vi "Upgrade Component Dependencies.vi"(0 "NIPKG_LV in":refnum<class "NIPKG_LV.lvclass">, 11 "error in (no error)":errorcluster) -> (4 "NIPKG_LV out":refnum<class "NIPKG_LV.lvclass">, 15 "error out":errorcluster)   [LabVIEW 2017, in "CL_G3_VIComponentBuilder.lvlib" / "NIPKG_LV.lvclass"]
doc: "Upgrades the NI Package versions that this NI Packages depends on. Adds the upgraded version information to the release notes."
uses:
  NIPKG_LV.lvclass
  C:/Tool Chain Support/Software Module Builder/Source/Exports/NI Build Specification_LV/NI Build Specification_LV.lvclass
  C:/Tool Chain Support/Software Module Builder/Source/Exports/Exports/Export.lvclass
  NI Build Specification_LV/NI Build Specification_LV.lvclass/NI Build Specification_LV.ctl
  <userlib>/_Cirrus Logic/NI Package Manager API/Source/Version Comparison Operator.ctl
  <vilib>/Utility/error.llb/whitespace.ctl
  Exports/Export.lvclass/Export.ctl
  NI Build Specification_LV/Accessors/Read Project Reference.vi
  NI Build Specification_LV/Accessors/Read Build Spec Ref.vi
  Exports/Accessors/Write Export Operation Errors.vi
  <userlib>/_Cirrus Logic/NI Package Manager API/Source/TCS_NIPKG_API.lvlib
  <userlib>/_Cirrus Logic/NI Package Manager BldSpec Utils/Source/NIPKG BuildSpec API.lvlib
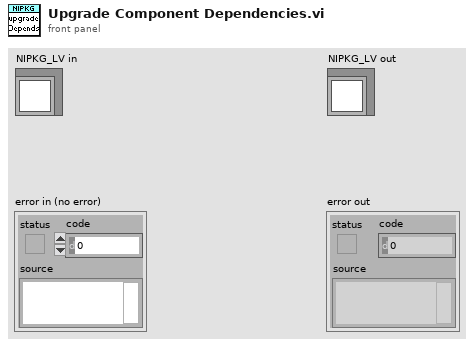
[diagram p1: front panel]
types:
  T1 = cluster{"NIPKG_LV":refnum<class "NIPKG_LV.lvclass">, "Upgrade Info":string[], "Release Notes":string, "Errors":errorcluster, "Release Notes Tag Name":string}
  T2 = typedef "TCS_NIPKG_API.lvlib/Version Comparison Operator.ctl" = enum16{">", ">=", "=", "!=", "<=", "<"}
  T3 = typedef "whitespace.ctl" = u16
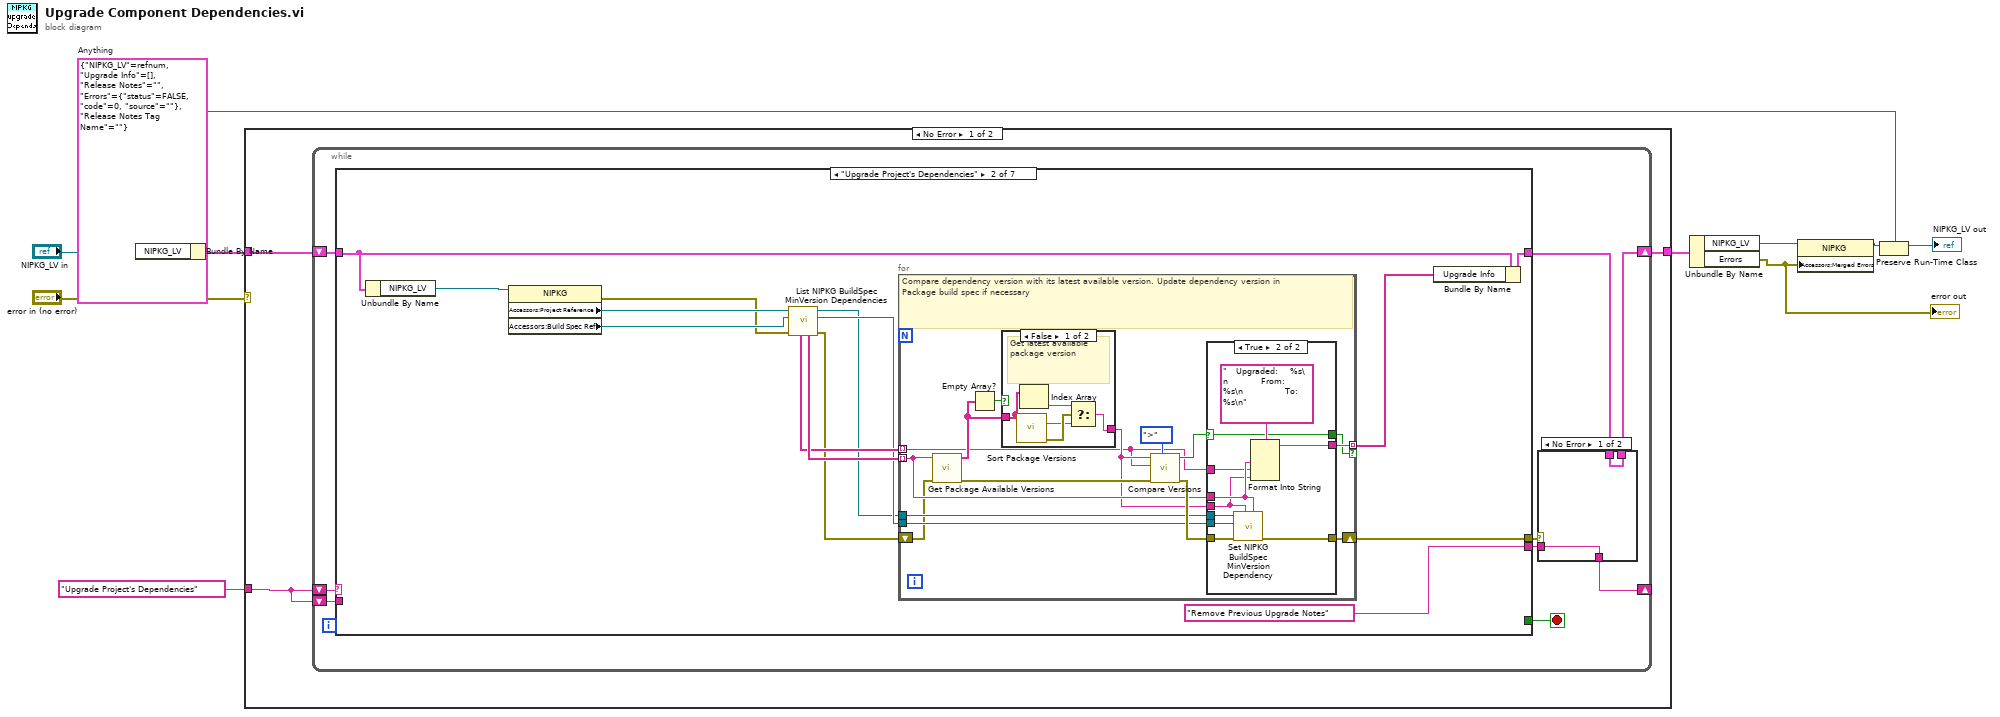
[diagram p0: block diagram]
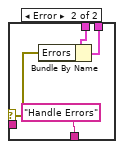
[diagram p2: hidden frame]
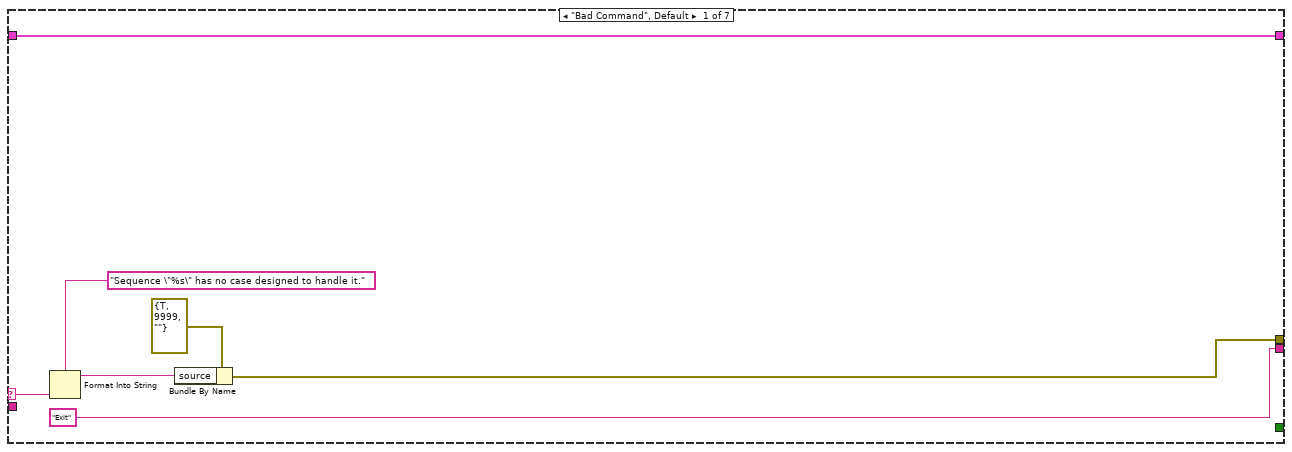
[diagram p3: hidden frame]
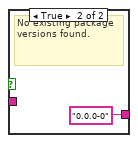
[diagram p4: hidden frame]
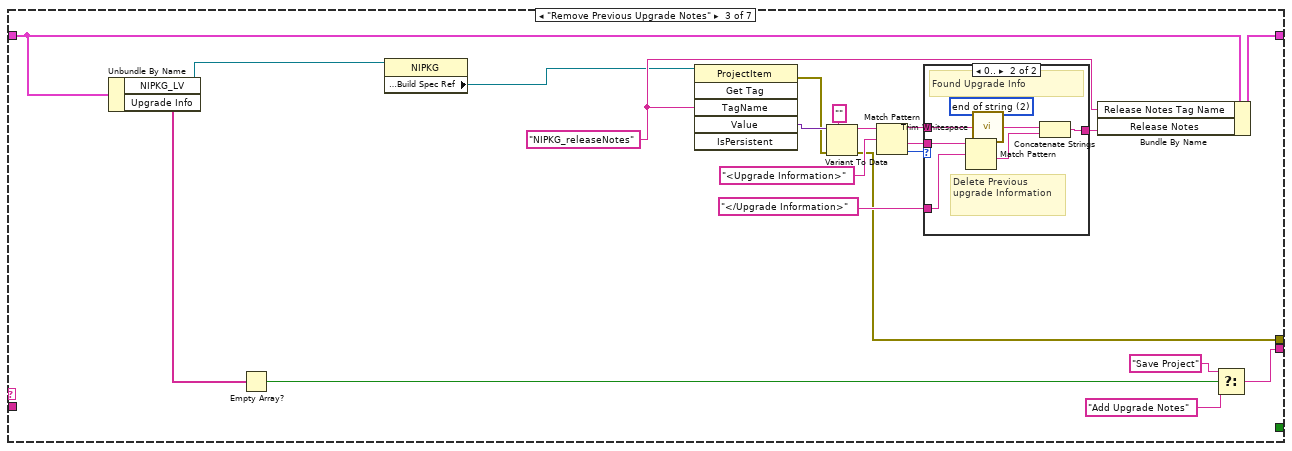
[diagram p6: hidden frame]
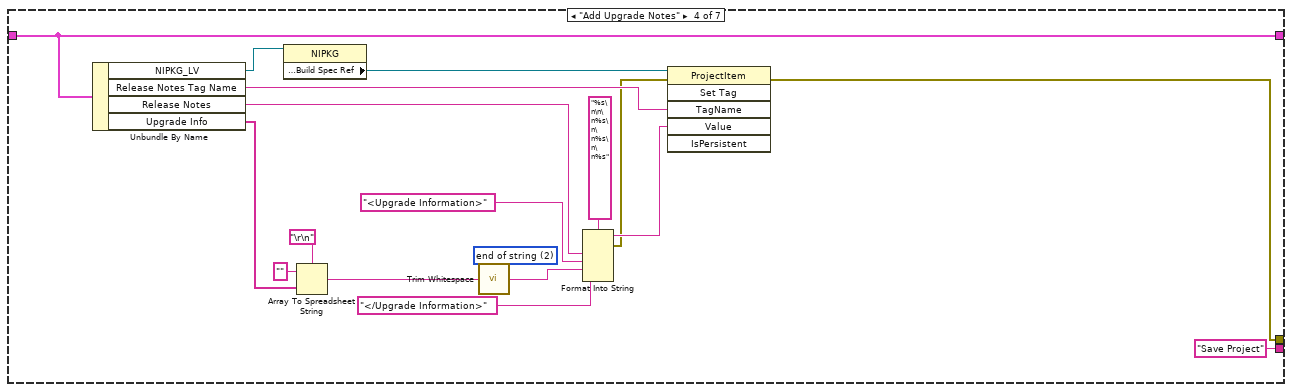
[diagram p8: hidden frame]
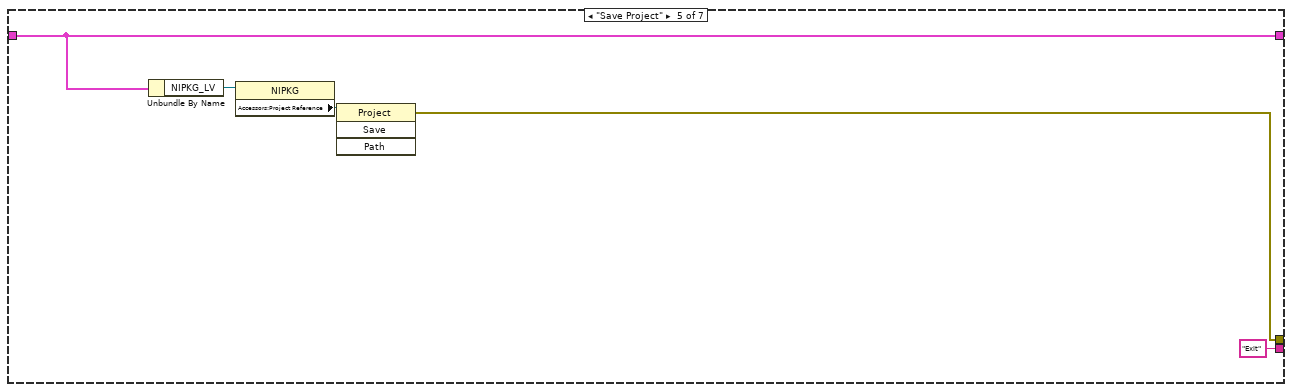
[diagram p9: hidden frame]
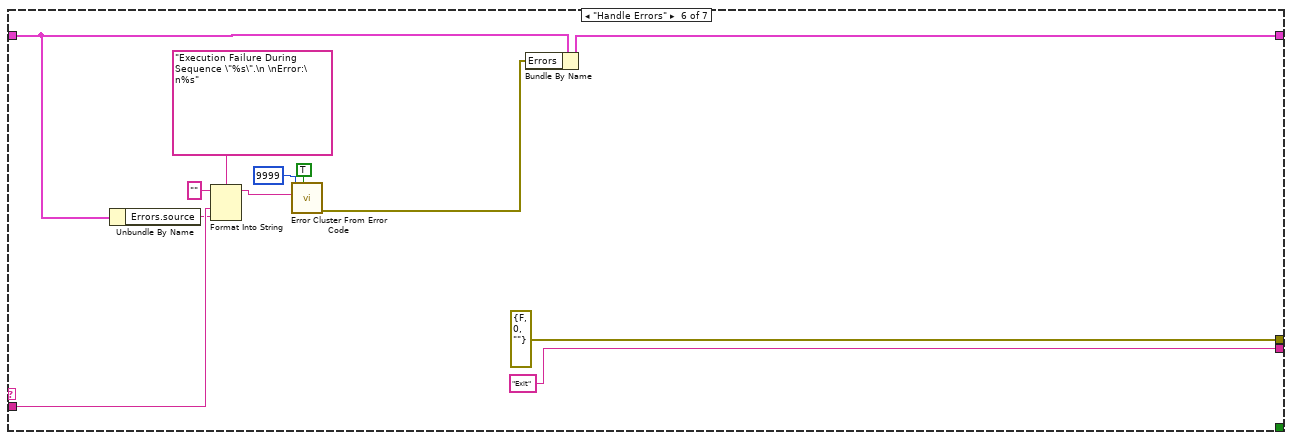
[diagram p10: hidden frame]
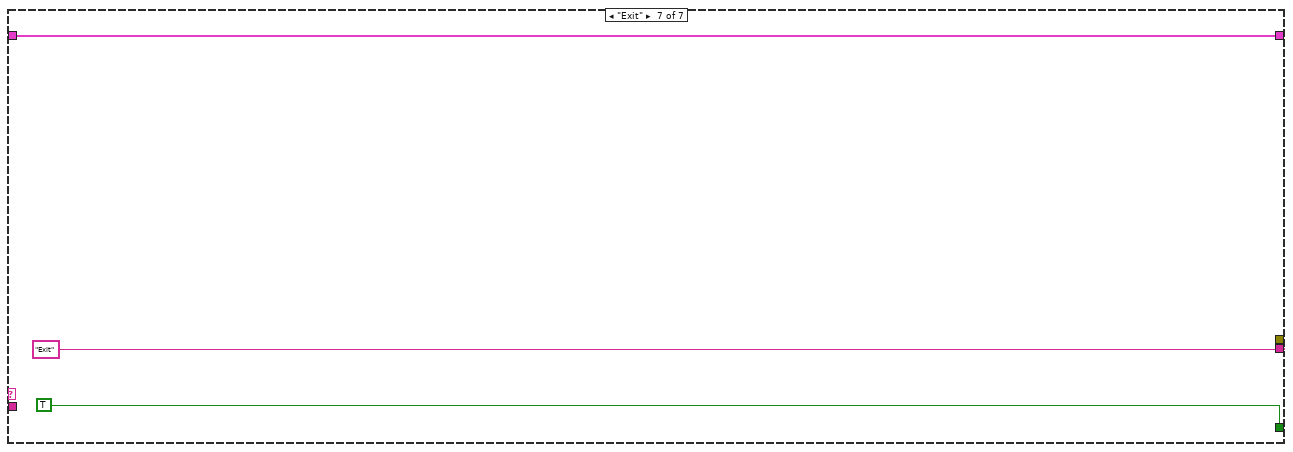
[diagram p11: hidden frame]
diagram:
  w8 = T1 {"NIPKG_LV"=refnum, "Upgrade Info"=[], "Release Notes"="", "Errors"={"status"=FALSE, "code"=0, "source"=""}, "Release Notes Tag Name"=""}  # Anything
  n1 = Bundle By Name(cluster=w8, "NIPKG_LV"="NIPKG_LV in") -> (w10:T1)
  n2 = case shown="No Error" "error in (no error)" {
    tunnel: "Upgrade Project's Dependencies" -> [w11 _]
    tunnel: w10 -> [w13 w149]
    tunnel: [w12 w149] -> w9
    frame No Error {
      n3 = while {
        shift-right: [w14] -> w12
        shift-left: w13 -> [w21]
        shift-right: [w19] -> _
        shift-left: w11 -> [w22]
        shift-left: w11 -> [w17]
        stop <- w16 stop-if-true
        n4 = case shown="\"Upgrade Project's Dependencies\"" w22 {
          selector: w22 -> [w29 _ _ _ _ _ _]
          tunnel: w21 -> [w35 w49 w95 w128 w133 w144 w148]
          tunnel: [w35 w41 w92 w128 w133 w137 w148] -> w15
          tunnel: [w33 w42 w89 w114 w132 errorcluster {"status"=FALSE, "code"=0, "source"=""} ("error out") _] -> w20
          tunnel: ["Exit" ("format string") "Remove Previous Upgrade Notes" ("format string") w87 "Save Project" ("format string") "Exit" ("format string") "Exit" ("format string") "Exit" ("format string")] -> w18
          tunnel: w17 -> [_ _ _ _ _ w135 _]
          tunnel: [_ _ _ _ _ _ TRUE] -> w16
          frame "Bad Command", Default {
            n5 = Format Into String(format string="Sequence \"%s\" has no case designed to handle it.", w29) -> (resulting string=w31:string)  [unwired: 2 in, 1 out]
            n6 = Bundle By Name(cluster=errorcluster {"status"=TRUE, "code"=9999, "source"=""} ("error out"), "source"=w31) -> (w33:errorcluster)
          }
          frame "Upgrade Project's Dependencies" {
            n7 = Unbundle By Name(w49) -> ("NIPKG_LV"=w48:refnum<class "NIPKG_LV.lvclass">)
            n8 = property class="NIPKG"(reference=w48) -> (error out=w36:errorcluster, "Accessors:Project Reference"=w38:refnum<vi>, "Accessors:Build Spec Ref"=w37:refnum<vi>)  [unwired: 1 in, 1 out]
            n9 = call <userlib>:"List NIPKG BuildSpec MinVersion Dependencies.vi"("error in (no error)"=w36, "package buildspec ref in"=w37, "project ref in"=w38) -> ("error out"=w44:errorcluster, "package buildspec ref out"=w45:refnum<vi>, "project ref out"=w43:refnum<vi>, "dependency package names"=w47:string[], "dependency package min versions"=w46:string[])  [unwired: 4 in]
            n10 = for {
              tunnel: w47 -> [w60] mode=indexing
              tunnel: w46 -> [w52] mode=indexing
              shift-right: [w56] -> w42
              shift-left: w44 -> [w57]
              tunnel: [w51] -> w40 mode=indexing if=w50
              tunnel: w43 -> [w59]
              tunnel: w45 -> [w58]
              # "Compare dependency version with its latest available version. Update dependency version in Package build spec if necessary"
              n11 = call <userlib>:"Get Package Available Versions.vi"("error in"=w57, "package name"=w60) -> ("error out"=w63:errorcluster, "Versions"=w53:string[])  [unwired: 8 in]
              n12 = Empty Array?(array=w53) -> (empty?=w55:bool)
              n13 = case shown="False" w55 {
                tunnel: w53 -> [w69 _]
                tunnel: [w65 "0.0.0-0" ("String")] -> w54
                frame False {
                  # "Get latest available package version"
                  n14 = call <userlib>:"Sort Package Versions.vi"("Package Versions"=w69) -> ("Newest Version"=w66:string, "error out"=w68:errorcluster)  [unwired: 11 in, 2 out]
                  n15 = Index Array(array=w69) -> (element=w67:string)  [unwired: 1 in]
                  n16 = Select(t=w67, s=w68, f=w66) -> (s? t:f=w65:string)
                }
                frame True {
                  # "No existing package versions found."
                }
              }
              n17 = call <userlib>:"Compare Versions.vi"("operator"=Version_Comparison_Operator.">", "error in"=w63, "version y"=w52, "version x"=w54) -> ("error out"=w61:errorcluster, "Satisfied?"=w62:bool)  [unwired: 6 in]
              n18 = case shown="True" w62 {
                selector: w62 -> [_ w72]
                tunnel: w61 -> [w71 w81]
                tunnel: w60 -> [_ w76]
                tunnel: w54 -> [_ w75]
                tunnel: w59 -> [_ w80]
                tunnel: w58 -> [_ w79]
                tunnel: [w71 w78] -> w56
                tunnel: w52 -> [_ w74]
                tunnel: [_ w73] -> w51
                tunnel: [_ w72] -> w50
                frame False {
                }
                frame True {
                  n19 = call <userlib>:"Set NIPKG BuildSpec MinVersion Dependency.vi"("dependency package name"=w76, "version"=w75, "error in (no error)"=w81, "package buildspec ref in"=w79, "project ref in"=w80) -> ("error out"=w78:errorcluster)  [unwired: 3 in, 3 out]
                  n20 = Format Into String(format string="   Upgraded:    %s\n           From:    %s\n              To:     %s\n", w76, w74, w75) -> (resulting string=w73:string)  [unwired: 2 in, 1 out]
                }
              }
            }
            n21 = Bundle By Name(cluster=w49, "Upgrade Info"=w40) -> (w41:T1)
          }
          frame "Remove Previous Upgrade Notes" {
            w83 = "NIPKG_releaseNotes" ("string")
            n22 = Unbundle By Name(w95) -> ("NIPKG_LV"=w94:refnum<class "NIPKG_LV.lvclass">, "Upgrade Info"=w86:string[])
            n23 = Empty Array?(array=w86) -> (empty?=w85:bool)
            n24 = property class="NIPKG"(reference=w94) -> ("Accessors:Build Spec Ref"=w82:refnum<vi>)  [unwired: 1 in, 2 out]
            n25 = invoke class="ProjectItem" method="Get Tag"(reference=w82, "TagName"=w83) -> (error out=w93:errorcluster, "Value"=w102:variant)  [unwired: 4 in, 4 out]
            n26 = Variant To Data(error in=w93, type="", Variant=w102) -> (data=w98:string, error out=w89:errorcluster)
            n27 = Match Pattern(string=w98, regular expression="<Upgrade Information>" ("format string")) -> (before substring=w99:string, after substring=w100:string, offset past match=w96:i32)  [unwired: 1 in, 1 out]
            n28 = case shown="0.." w96 {
              tunnel: w100 -> [_ w110]
              tunnel: w99 -> [w103 w107]
              tunnel: [w103 w105] -> w91
              tunnel: "</Upgrade Information>" ("format string") -> [_ w104]
              frame Default {
                # "No Upgrade Info Found"
              }
              frame 0.. {
                w108 = T3 2 items=["both", "start of string", "end of string"] ("location (both)")
                # "Delete Previous upgrade Information"
                # "Found Upgrade Info"
                n29 = Match Pattern(string=w110, regular expression=w104) -> (after substring=w109:string)  [unwired: 1 in, 3 out]
                n30 = call <vilib>:"Trim Whitespace.vi"("string"=w107, "location (both)"=w108) -> ("trimmed string"=w106:string)
                n31 = Concatenate Strings(w106, w109) -> (w105:string)
              }
            }
            n32 = Bundle By Name(cluster=w95, "Release Notes Tag Name"=w83, "Release Notes"=w91) -> (w92:T1)
            n33 = Select(t="Save Project" ("format string"), s=w85, f="Add Upgrade Notes" ("format string")) -> (s? t:f=w87:string)
          }
          frame "Add Upgrade Notes" {
            w123 = T3 2 items=["both", "start of string", "end of string"] ("location (both)")
            n34 = Unbundle By Name(w128) -> ("NIPKG_LV"=w112:refnum<class "NIPKG_LV.lvclass">, "Release Notes Tag Name"=w115:string, "Release Notes"=w116:string, "Upgrade Info"=w125:string[])
            n35 = property class="NIPKG"(reference=w112) -> ("Accessors:Build Spec Ref"=w111:refnum<vi>)  [unwired: 1 in, 2 out]
            n36 = Array To Spreadsheet String(delimiter (Tab)="\r\n", array=w125, 3:"" ("format string")) -> (spreadsheet string=w126:string)
            n37 = call <vilib>:"Trim Whitespace.vi"("string"=w126, "location (both)"=w123) -> ("trimmed string"=w119:string)
            n38 = Format Into String(format string="%s\n\n\n%s\n\n%s\n\n%s", w116, "<Upgrade Information>" ("format string"), w119, "</Upgrade Information>" ("format string")) -> (resulting string=w118:string, error out=w113:errorcluster)  [unwired: 2 in]
            n39 = invoke class="ProjectItem" method="Set Tag"(reference=w111, error in=w113, "TagName"=w115, "Value"=w118) -> (error out=w114:errorcluster)  [unwired: 2 in, 5 out]
          }
          frame "Save Project" {
            n40 = Unbundle By Name(w133) -> ("NIPKG_LV"=w130:refnum<class "NIPKG_LV.lvclass">)
            n41 = property class="NIPKG"(reference=w130) -> ("Accessors:Project Reference"=w129:refnum<vi>)  [unwired: 1 in, 2 out]
            n42 = invoke class="Project" method="Save"(reference=w129) -> (error out=w132:errorcluster)  [unwired: 3 in, 3 out]
          }
          frame "Handle Errors" {
            n43 = Unbundle By Name(w144) -> ("Errors.source"=w134:string)
            n44 = Format Into String(format string="Execution Failure During Sequence \"%s\".\n \nError:\n%s" ("error message (\"\")"), initial string="", w135, w134) -> (resulting string=w141:string)  [unwired: 1 in, 1 out]
            n45 = call <vilib>:"Error Cluster From Error Code.vi"("show call chain? (False)"=TRUE, "error message (\"\")"=w141, "error code (0)"=9999) -> ("error out"=w136:errorcluster)  [unwired: 6 in]
            n46 = Bundle By Name(cluster=w144, "Errors"=w136) -> (w137:T1)
          }
          frame "Exit" {
          }
        }
        n47 = case shown="No Error" w20 {
          selector: w20 -> [_ w28]
          tunnel: [w23 "Handle Errors"] -> w19
          tunnel: w18 -> [w23 _]
          tunnel: w15 -> [w24 w27]
          tunnel: [w24 w26] -> w14
          frame No Error {
          }
          frame Error {
            n48 = Bundle By Name(cluster=w27, "Errors"=w28) -> (w26:T1)
          }
        }
      }
    }
    frame Error {
    }
  }
  n49 = Unbundle By Name(w9) -> ("NIPKG_LV"=w5:refnum<class "NIPKG_LV.lvclass">, "Errors"=w1:errorcluster)
  "error out" <- w1
  n50 = property class="NIPKG"(reference=w5, "Accessors:Merged Errors"=w1) -> (reference out=w4:refnum<class "NIPKG_LV.lvclass">)  [unwired: 1 in, 1 out]
  n51 = Preserve Run-Time Class(object in=w4, 2:"NIPKG_LV in") -> (object out=→"NIPKG_LV out":refnum<class "NIPKG_LV.lvclass">)  [unwired: 1 in, 1 out]
